vi "Defaults.vi"(8 "error in (no error)":errorcluster, 11 "MB Slave in":refnum<class "iC7-AFE.lvclass">) -> (0 "error out":errorcluster, 3 "MB Slave out":refnum<class "iC7-AFE.lvclass">)   [LabVIEW 2021, in "iC7-AFE.lvclass"]
uses:
  iC7-AFE.lvclass
  C:/Program Files (x86)/National Instruments/LabVIEW 2021/user.lib/S2 Labs/Module Framework/Modules/Base/Module.lvclass
  C:/Program Files (x86)/National Instruments/LabVIEW 2021/user.lib/S2 Labs/Module Framework/Modules/Modbus/Modbus Slave Base/Modbus Slave Base.lvclass
  <userlib>/S2 Labs/Module Framework/Modules/Base/Module.lvclass/Module.ctl
  <userlib>/S2 Labs/Modbus Toolkit/TypeDefs/MB Element.ctl
  <userlib>/S2 Labs/Modbus Toolkit/TypeDefs/Endianness Type.ctl
  <userlib>/S2 Labs/Modbus Toolkit/TypeDefs/Access Type.ctl
  <userlib>/S2 Labs/Module Framework/Modules/Modbus/Modbus Slave Base/Modbus Slave Base.lvclass/Modbus Slave Base.ctl
  <userlib>/S2 Labs/Module Framework/Modules/Base/Read Name.vi
  <userlib>/S2 Labs/Module Framework/Modules/Modbus/Modbus Slave Base/Write MB Map.vi
  MB Slave Simulator Base/MB Slave Simulator Base.lvclass
  <userlib>/S2 Labs/Modbus Toolkit/S2L Modbus API.lvclass
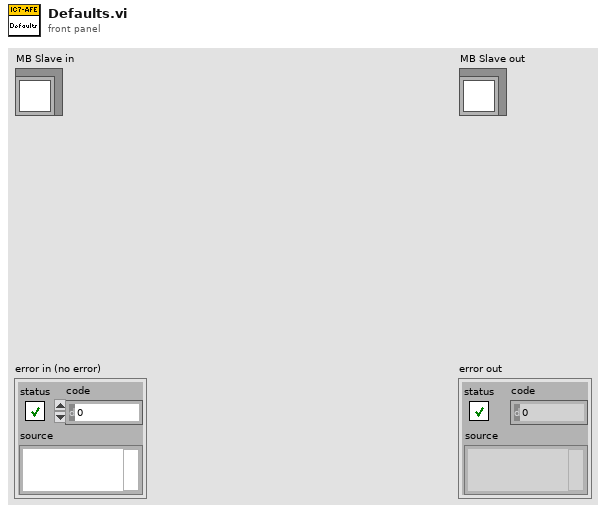
[diagram p1: front panel]
types:
  T1 = typedef "S2L Modbus API.lvclass/MB Element.ctl" = cluster{"Label":string, "Prefix":u8, "Address":u16, "Datatype":string, "Register Count":u8, "Multiplier":dbl, "Offset":dbl, "Unit":string, "Endianness":T2, "Access":T3, "LUT":string[], "Poll Rate(ms)":u16, "Mapping":cluster{"Module":string, "Channel":string}}
  T2 = typedef "Endianness Type.ctl" = enum16{"Big-Endian", "Little-Endian", "Big-Endian Byte Swap", "Little-Endian Byte Swap"}
  T3 = typedef "S2L Modbus API.lvclass/Access Type.ctl" = enum16{"R/W", "R", "W"}
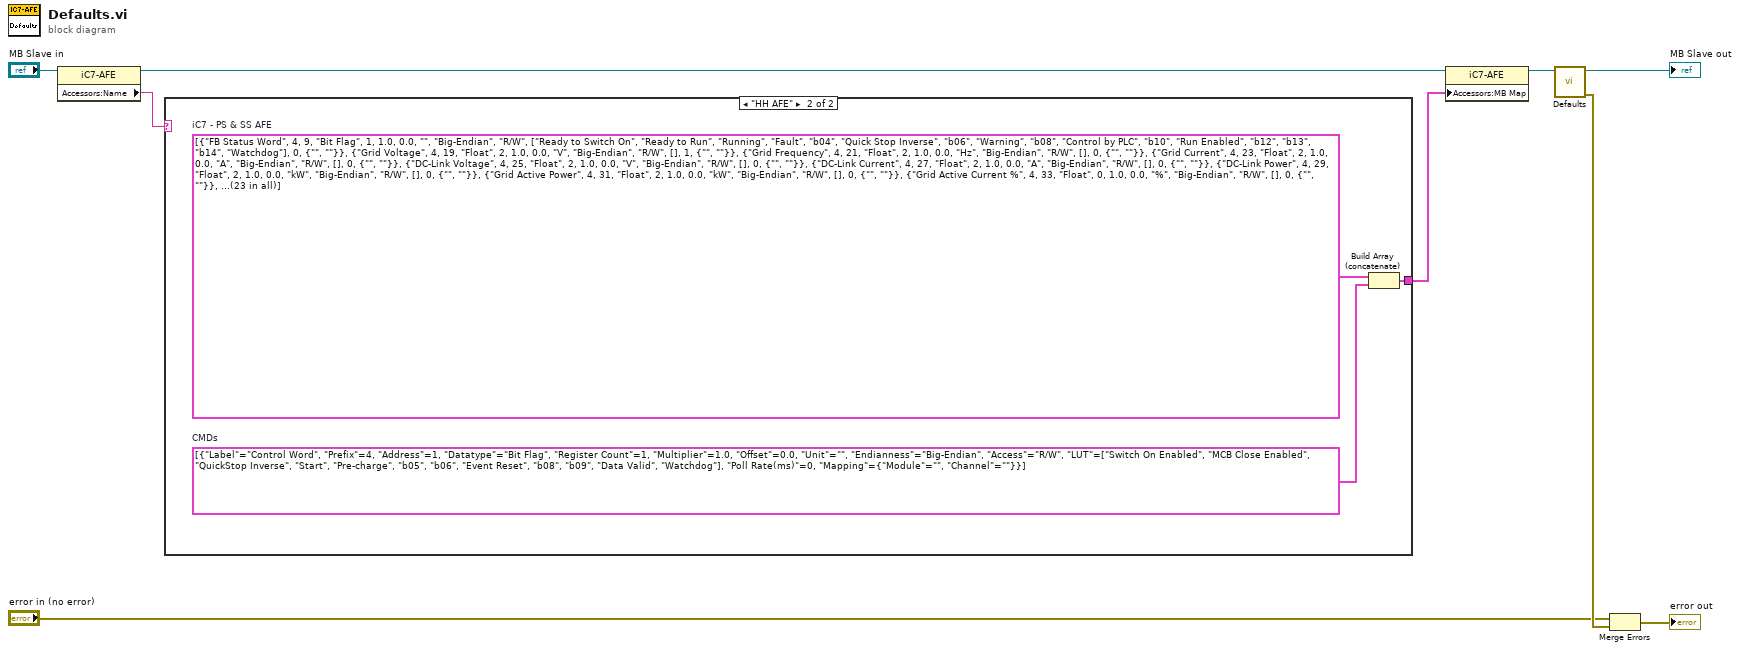
[diagram p0: block diagram]
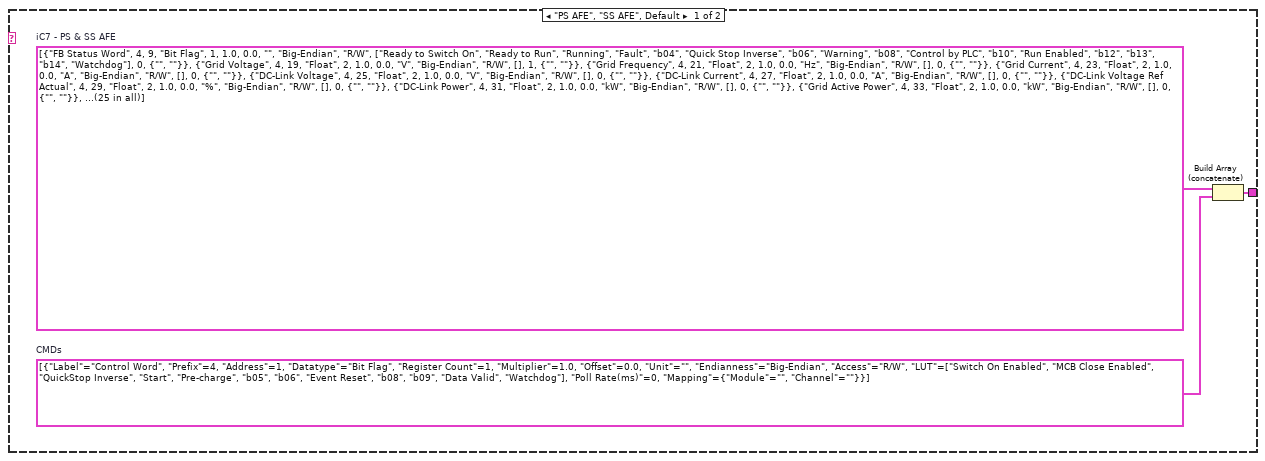
[diagram p2: hidden frame]
diagram:
  n1 = property class="iC7-AFE"(reference="MB Slave in") -> (reference out=w6:refnum<class "iC7-AFE.lvclass">, "Accessors:Name"=w1:string)  [unwired: 1 in, 1 out]
  n2 = case shown="\"HH AFE\"" w1 {
    tunnel: [w11 w14] -> w2
    frame "PS AFE", "SS AFE", Default {
      w10 = T1[] [{"Label"="Control Word", "Prefix"=4, "Address"=1, "Datatype"="Bit Flag", "Register Count"=1, "Multiplier"=1.0, "Offset"=0.0, "Unit"="", "Endianness"=enum."Big-Endian", "Access"=enum."R/W", "LUT"=["Switch On Enabled", "MCB Close Enabled", "QuickStop Inverse", "Start", "Pre-charge", "b05", "b06", "Event Reset", "b08", "b09", "Data Valid", "Watchdog"], "Poll Rate(ms)"=0, "Mapping"={"Module"="", "Channel"=""}}]  # CMDs
      w12 = T1[] [{"Label"="FB Status Word", "Prefix"=4, "Address"=9, "Datatype"="Bit Flag", "Register Count"=1, "Multiplier"=1.0, "Offset"=0.0, "Unit"="", "Endianness"=enum."Big-Endian", "Access"=enum."R/W", "LUT"=["Ready to Switch On", "Ready to Run", "Running", "Fault", "b04", "Quick Stop Inverse", "b06", "Warning", "b08", "Control by PLC", "b10", "Run Enabled", "b12", "b13", "b14", "Watchdog"], "Poll Rate(ms)"=0, "Mapping"={"Module"="", "Channel"=""}}, {"Label"="Grid Voltage", "Prefix"=4, "Address"=19, "Datatype"="Float", "Register Count"=2, "Multiplier"=1.0, "Offset"=0.0, "Unit"="V", "Endianness"=enum."Big-Endian", "Access"=enum."R/W", "LUT"=[], "Poll Rate(ms)"=1, "Mapping"={"Module"="", "Channel"=""}}, {"Label"="Grid Frequency", "Prefix"=4, "Address"=21, "Datatype"="Float", "Register Count"=2, "Multiplier"=1.0, "Offset"=0.0, "Unit"="Hz", "Endianness"=enum."Big-Endian", "Access"=enum."R/W", "LUT"=[], "Poll Rate(ms)"=0, "Mapping"={"Module"="", "Channel"=""}}, {"Label"="Grid Current", "Prefix"=4, "Address"=23, "Datatype"="Float", "Register Count"=2, "Multiplier"=1.0, "Offset"=0.0, "Unit"="A", "Endianness"=enum."Big-Endian", "Access"=enum."R/W", "LUT"=[], "Poll Rate(ms)"=0, "Mapping"={"Module"="", "Channel"=""}}, {"Label"="DC-Link Voltage", "Prefix"=4, "Address"=25, "Datatype"="Float", "Register Count"=2, "Multiplier"=1.0, "Offset"=0.0, "Unit"="V", "Endianness"=enum."Big-Endian", "Access"=enum."R/W", "LUT"=[], "Poll Rate(ms)"=0, "Mapping"={"Module"="", "Channel"=""}}, {"Label"="DC-Link Current", "Prefix"=4, "Address"=27, "Datatype"="Float", "Register Count"=2, "Multiplier"=1.0, "Offset"=0.0, "Unit"="A", "Endianness"=enum."Big-Endian", "Access"=enum."R/W", "LUT"=[], "Poll Rate(ms)"=0, "Mapping"={"Module"="", "Channel"=""}}, {"Label"="DC-Link Voltage Ref Actual", "Prefix"=4, "Address"=29, "Datatype"="Float", "Register Count"=2, "Multiplier"=1.0, "Offset"=0.0, "Unit"="%", "Endianness"=enum."Big-Endian", "Access"=enum."R/W", "LUT"=[], "Poll Rate(ms)"=0, "Mapping"={"Module"="", "Channel"=""}}, {"Label"="DC-Link Power", "Prefix"=4, "Address"=31, "Datatype"="Float", "Register Count"=2, "Multiplier"=1.0, "Offset"=0.0, "Unit"="kW", "Endianness"=enum."Big-Endian", "Access"=enum."R/W", "LUT"=[], "Poll Rate(ms)"=0, "Mapping"={"Module"="", "Channel"=""}}, {"Label"="Grid Active Power", "Prefix"=4, "Address"=33, "Datatype"="Float", "Register Count"=2, "Multiplier"=1.0, "Offset"=0.0, "Unit"="kW", "Endianness"=enum."Big-Endian", "Access"=enum."R/W", "LUT"=[], "Poll Rate(ms)"=0, "Mapping"={"Module"="", "Channel"=""}}, {"Label"="Grid Active Current %", "Prefix"=4, "Address"=35, "Datatype"="Float", "Register Count"=2, "Multiplier"=1.0, "Offset"=0.0, "Unit"="%", "Endianness"=enum."Big-Endian", "Access"=enum."R/W", "LUT"=[], "Poll Rate(ms)"=0, "Mapping"={"Module"="", "Channel"=""}}, {"Label"="Grid Reactive Current %", "Prefix"=4, "Address"=37, "Datatype"="Float", "Register Count"=2, "Multiplier"=1.0, "Offset"=0.0, "Unit"="%", "Endianness"=enum."Big-Endian", "Access"=enum."R/W", "LUT"=[], "Poll Rate(ms)"=0, "Mapping"={"Module"="", "Channel"=""}}, {"Label"="Grid Power Factor", "Prefix"=4, "Address"=39, "Datatype"="Float", "Register Count"=2, "Multiplier"=1.0, "Offset"=0.0, "Unit"="", "Endianness"=enum."Big-Endian", "Access"=enum."R/W", "LUT"=[], "Poll Rate(ms)"=0, "Mapping"={"Module"="", "Channel"=""}}, {"Label"="Fault Status Word 1", "Prefix"=4, "Address"=41, "Datatype"="Bit Flag", "Register Count"=1, "Multiplier"=1.0, "Offset"=0.0, "Unit"="", "Endianness"=enum."Big-Endian", "Access"=enum."R/W", "LUT"=["Over current", "DC-Link Over voltage", "DC-Link Under voltage", "b03-Reserved", "Unit under temperature", "b05-Reserved", "b06-Reserved", "b07-Reserved", "Earth Fault", "b09-Reserved", "Fieldbus issue", "HMI control lost", "b12-Reserved", "Thermistor Fault", "Auxiliary device", "External temperature measurement"], "Poll Rate(ms)"=0, "Mapping"={"Module"="", "Channel"=""}}, {"Label"="Fault Status Word 2", "Prefix"=4, "Address"=42, "Datatype"="Bit Flag", "Register Count"=1, "Multiplier"=1.0, "Offset"=0.0, "Unit"="", "Endianness"=enum."Big-Endian", "Access"=enum."R/W", "LUT"=["Analog Input Live Zero", "Pre charge Failed", "MCB Feedback Fault", "Quick Stop Active", "Thermistor Over Temperature", "MCB Trip", "External Fault", "Cooling Supervision Fault", "Fieldbus Watchdog", "Line Synchronization Fault", "Short Term Current Injection"], "Poll Rate(ms)"=0, "Mapping"={"Module"="", "Channel"=""}}, {"Label"="Warning Status Word 1", "Prefix"=4, "Address"=43, "Datatype"="Bit Flag", "Register Count"=1, "Multiplier"=1.0, "Offset"=0.0, "Unit"="", "Endianness"=enum."Big-Endian", "Access"=enum."R/W", "LUT"=["Over current", "DC-Link Over voltage", "DC-Link Under voltage", "b03-Reserved", "Unit under temperature ", "b05-Reserved", "b06-Reserved", "b07-Reserved", "Earth Warning", "b09-Reserved", "Fieldbus issue", "HMI control lost", "b12-Reserved", "Thermistor Warning", "Auxiliary device", "External temperature measurement"], "Poll Rate(ms)"=0, "Mapping"={"Module"="", "Channel"=""}}, {"Label"="Warning Status Word 2", "Prefix"=4, "Address"=44, "Datatype"="Bit Flag", "Register Count"=1, "Multiplier"=1.0, "Offset"=0.0, "Unit"="", "Endianness"=enum."Big-Endian", "Access"=enum."R/W", "LUT"=["Analog Input Live Zero", "b01-Reserved", "b02-Reserved", "Quick Stop Active", "Thermistor Over Temperature", "b05-Reserved", "External Warning", "Cooling Supervision Warning", "Fieldbus Watchdog", "b09-Reserved", "Short Term Current Injection"], "Poll Rate(ms)"=0, "Mapping"={"Module"="", "Channel"=""}}, {"Label"="DI Bit Word", "Prefix"=4, "Address"=45, "Datatype"="Bit Flag", "Register Count"=1, "Multiplier"=1.0, "Offset"=0.0, "Unit"="", "Endianness"=enum."Big-Endian", "Access"=enum."R/W", "LUT"=["b00", "b01", "b02", "Breaker Charged", "b04", "b05", "b06", "b07", "b08", "b09", "b10", "b11", "b12", "b13", "b14", "b15"], "Poll Rate(ms)"=0, "Mapping"={"Module"="", "Channel"=""}}, {"Label"="DO Bit Word", "Prefix"=4, "Address"=46, "Datatype"="Bit Flag", "Register Count"=1, "Multiplier"=1.0, "Offset"=0.0, "Unit"="", "Endianness"=enum."Big-Endian", "Access"=enum."R/W", "LUT"=["b00", "b01", "b02", "b03", "b04", "b05", "b06", "b07", "b08", "b09", "b10", "b11", "b12", "b13", "b14", "b15"], "Poll Rate(ms)"=0, "Mapping"={"Module"="", "Channel"=""}}, {"Label"="PreCharge Active", "Prefix"=4, "Address"=47, "Datatype"="U16", "Register Count"=1, "Multiplier"=1.0, "Offset"=0.0, "Unit"="", "Endianness"=enum."Big-Endian", "Access"=enum."R/W", "LUT"=[], "Poll Rate(ms)"=0, "Mapping"={"Module"="", "Channel"=""}}, {"Label"="MCB Feedback", "Prefix"=4, "Address"=48, "Datatype"="U16", "Register Count"=1, "Multiplier"=1.0, "Offset"=0.0, "Unit"="", "Endianness"=enum."Big-Endian", "Access"=enum."R/W", "LUT"=[], "Poll Rate(ms)"=0, "Mapping"={"Module"="", "Channel"=""}}, {"Label"="Heatsink Unit Temp", "Prefix"=4, "Address"=49, "Datatype"="Float", "Register Count"=2, "Multiplier"=1.0, "Offset"=0.0, "Unit"="C", "Endianness"=enum."Big-Endian", "Access"=enum."R/W", "LUT"=[], "Poll Rate(ms)"=0, "Mapping"={"Module"="", "Channel"=""}}, {"Label"="Grid Nominal Power", "Prefix"=4, "Address"=51, "Datatype"="Float", "Register Count"=2, "Multiplier"=1.0, "Offset"=0.0, "Unit"="kVA", "Endianness"=enum."Big-Endian", "Access"=enum."R/W", "LUT"=[], "Poll Rate(ms)"=0, "Mapping"={"Module"="", "Channel"=""}}, {"Label"="DC-Link Voltage Ref", "Prefix"=4, "Address"=53, "Datatype"="Float", "Register Count"=2, "Multiplier"=1.0, "Offset"=0.0, "Unit"="V", "Endianness"=enum."Big-Endian", "Access"=enum."R/W", "LUT"=[], "Poll Rate(ms)"=0, "Mapping"={"Module"="", "Channel"=""}}, {"Label"="DC-Link Voltage Ramp Rate", "Prefix"=4, "Address"=55, "Datatype"="Float", "Register Count"=2, "Multiplier"=1.0, "Offset"=0.0, "Unit"="percent/sec", "Endianness"=enum."Big-Endian", "Access"=enum."R/W", "LUT"=[], "Poll Rate(ms)"=0, "Mapping"={"Module"="", "Channel"=""}}, {"Label"="FB Active Power Ref", "Prefix"=4, "Address"=57, "Datatype"="Float", "Register Count"=2, "Multiplier"=1.0, "Offset"=0.0, "Unit"="kW", "Endianness"=enum."Big-Endian", "Access"=enum."R/W", "LUT"=[], "Poll Rate(ms)"=0, "Mapping"={"Module"="", "Channel"=""}}]  # iC7 - PS & SS AFE
      n3 = Build Array (concatenate)(w12, w10) -> (w11:T1[])
    }
    frame "HH AFE" {
      w13 = T1[] [{"Label"="Control Word", "Prefix"=4, "Address"=1, "Datatype"="Bit Flag", "Register Count"=1, "Multiplier"=1.0, "Offset"=0.0, "Unit"="", "Endianness"=enum."Big-Endian", "Access"=enum."R/W", "LUT"=["Switch On Enabled", "MCB Close Enabled", "QuickStop Inverse", "Start", "Pre-charge", "b05", "b06", "Event Reset", "b08", "b09", "Data Valid", "Watchdog"], "Poll Rate(ms)"=0, "Mapping"={"Module"="", "Channel"=""}}]  # CMDs
      w15 = T1[] [{"Label"="FB Status Word", "Prefix"=4, "Address"=9, "Datatype"="Bit Flag", "Register Count"=1, "Multiplier"=1.0, "Offset"=0.0, "Unit"="", "Endianness"=enum."Big-Endian", "Access"=enum."R/W", "LUT"=["Ready to Switch On", "Ready to Run", "Running", "Fault", "b04", "Quick Stop Inverse", "b06", "Warning", "b08", "Control by PLC", "b10", "Run Enabled", "b12", "b13", "b14", "Watchdog"], "Poll Rate(ms)"=0, "Mapping"={"Module"="", "Channel"=""}}, {"Label"="Grid Voltage", "Prefix"=4, "Address"=19, "Datatype"="Float", "Register Count"=2, "Multiplier"=1.0, "Offset"=0.0, "Unit"="V", "Endianness"=enum."Big-Endian", "Access"=enum."R/W", "LUT"=[], "Poll Rate(ms)"=1, "Mapping"={"Module"="", "Channel"=""}}, {"Label"="Grid Frequency", "Prefix"=4, "Address"=21, "Datatype"="Float", "Register Count"=2, "Multiplier"=1.0, "Offset"=0.0, "Unit"="Hz", "Endianness"=enum."Big-Endian", "Access"=enum."R/W", "LUT"=[], "Poll Rate(ms)"=0, "Mapping"={"Module"="", "Channel"=""}}, {"Label"="Grid Current", "Prefix"=4, "Address"=23, "Datatype"="Float", "Register Count"=2, "Multiplier"=1.0, "Offset"=0.0, "Unit"="A", "Endianness"=enum."Big-Endian", "Access"=enum."R/W", "LUT"=[], "Poll Rate(ms)"=0, "Mapping"={"Module"="", "Channel"=""}}, {"Label"="DC-Link Voltage", "Prefix"=4, "Address"=25, "Datatype"="Float", "Register Count"=2, "Multiplier"=1.0, "Offset"=0.0, "Unit"="V", "Endianness"=enum."Big-Endian", "Access"=enum."R/W", "LUT"=[], "Poll Rate(ms)"=0, "Mapping"={"Module"="", "Channel"=""}}, {"Label"="DC-Link Current", "Prefix"=4, "Address"=27, "Datatype"="Float", "Register Count"=2, "Multiplier"=1.0, "Offset"=0.0, "Unit"="A", "Endianness"=enum."Big-Endian", "Access"=enum."R/W", "LUT"=[], "Poll Rate(ms)"=0, "Mapping"={"Module"="", "Channel"=""}}, {"Label"="DC-Link Power", "Prefix"=4, "Address"=29, "Datatype"="Float", "Register Count"=2, "Multiplier"=1.0, "Offset"=0.0, "Unit"="kW", "Endianness"=enum."Big-Endian", "Access"=enum."R/W", "LUT"=[], "Poll Rate(ms)"=0, "Mapping"={"Module"="", "Channel"=""}}, {"Label"="Grid Active Power", "Prefix"=4, "Address"=31, "Datatype"="Float", "Register Count"=2, "Multiplier"=1.0, "Offset"=0.0, "Unit"="kW", "Endianness"=enum."Big-Endian", "Access"=enum."R/W", "LUT"=[], "Poll Rate(ms)"=0, "Mapping"={"Module"="", "Channel"=""}}, {"Label"="Grid Active Current %", "Prefix"=4, "Address"=33, "Datatype"="Float", "Register Count"=0, "Multiplier"=1.0, "Offset"=0.0, "Unit"="%", "Endianness"=enum."Big-Endian", "Access"=enum."R/W", "LUT"=[], "Poll Rate(ms)"=0, "Mapping"={"Module"="", "Channel"=""}}, {"Label"="Grid Reactive Current %", "Prefix"=4, "Address"=35, "Datatype"="Float", "Register Count"=0, "Multiplier"=1.0, "Offset"=0.0, "Unit"="%", "Endianness"=enum."Big-Endian", "Access"=enum."R/W", "LUT"=[], "Poll Rate(ms)"=0, "Mapping"={"Module"="", "Channel"=""}}, {"Label"="Grid Power Factor", "Prefix"=4, "Address"=37, "Datatype"="Float", "Register Count"=0, "Multiplier"=1.0, "Offset"=0.0, "Unit"="", "Endianness"=enum."Big-Endian", "Access"=enum."R/W", "LUT"=[], "Poll Rate(ms)"=0, "Mapping"={"Module"="", "Channel"=""}}, {"Label"="Fault Status Word 1", "Prefix"=4, "Address"=39, "Datatype"="Bit Flag", "Register Count"=0, "Multiplier"=1.0, "Offset"=0.0, "Unit"="", "Endianness"=enum."Big-Endian", "Access"=enum."R/W", "LUT"=["Over current", "DC-Link Over voltage", "DC-Link Under voltage", "b03-Reserved", "Unit under temperature", "b05-Reserved", "b06-Reserved", "b07-Reserved", "Earth Fault", "b09-Reserved", "Fieldbus issue", "HMI control lost", "b12-Reserved", "Thermistor Fault", "Auxiliary device", "External temperature measurement"], "Poll Rate(ms)"=0, "Mapping"={"Module"="", "Channel"=""}}, {"Label"="Fault Status Word 2", "Prefix"=4, "Address"=40, "Datatype"="Bit Flag", "Register Count"=0, "Multiplier"=1.0, "Offset"=0.0, "Unit"="", "Endianness"=enum."Big-Endian", "Access"=enum."R/W", "LUT"=["Analog Input Live Zero", "Pre charge Failed", "MCB Feedback Fault", "Quick Stop Active", "Thermistor Over Temperature", "MCB Trip", "External Fault", "Cooling Supervision Fault", "Fieldbus Watchdog", "Line Synchronization Fault", "Short Term Current Injection"], "Poll Rate(ms)"=0, "Mapping"={"Module"="", "Channel"=""}}, {"Label"="Warning Status Word 1", "Prefix"=4, "Address"=41, "Datatype"="Bit Flag", "Register Count"=0, "Multiplier"=1.0, "Offset"=0.0, "Unit"="", "Endianness"=enum."Big-Endian", "Access"=enum."R/W", "LUT"=["Over current", "DC-Link Over voltage", "DC-Link Under voltage", "b03-Reserved", "Unit under temperature ", "b05-Reserved", "b06-Reserved", "b07-Reserved", "Earth Warning", "b09-Reserved", "Fieldbus issue", "HMI control lost", "b12-Reserved", "Thermistor Warning", "Auxiliary device", "External temperature measurement"], "Poll Rate(ms)"=0, "Mapping"={"Module"="", "Channel"=""}}, {"Label"="Warning Status Word 2", "Prefix"=4, "Address"=42, "Datatype"="Bit Flag", "Register Count"=0, "Multiplier"=1.0, "Offset"=0.0, "Unit"="", "Endianness"=enum."Big-Endian", "Access"=enum."R/W", "LUT"=["Analog Input Live Zero", "b01-Reserved", "b02-Reserved", "Quick Stop Active", "Thermistor Over Temperature", "b05-Reserved", "External Warning", "Cooling Supervision Warning", "Fieldbus Watchdog", "b09-Reserved", "Short Term Current Injection"], "Poll Rate(ms)"=0, "Mapping"={"Module"="", "Channel"=""}}, {"Label"="DI Bit Word", "Prefix"=4, "Address"=43, "Datatype"="Bit Flag", "Register Count"=0, "Multiplier"=1.0, "Offset"=0.0, "Unit"="", "Endianness"=enum."Big-Endian", "Access"=enum."R/W", "LUT"=["b00", "b01", "b02", "b03", "b04", "b05", "b06", "b07", "b08", "b09", "b10", "b11", "b12", "b13", "b14", "b15"], "Poll Rate(ms)"=0, "Mapping"={"Module"="", "Channel"=""}}, {"Label"="DO Bit Word", "Prefix"=4, "Address"=44, "Datatype"="Bit Flag", "Register Count"=0, "Multiplier"=1.0, "Offset"=0.0, "Unit"="", "Endianness"=enum."Big-Endian", "Access"=enum."R/W", "LUT"=["b00", "b01", "b02", "b03", "b04", "b05", "b06", "b07", "b08", "b09", "b10", "b11", "b12", "b13", "b14", "b15"], "Poll Rate(ms)"=0, "Mapping"={"Module"="", "Channel"=""}}, {"Label"="PreCharge Active", "Prefix"=4, "Address"=45, "Datatype"="U16", "Register Count"=0, "Multiplier"=1.0, "Offset"=0.0, "Unit"="", "Endianness"=enum."Big-Endian", "Access"=enum."R/W", "LUT"=[], "Poll Rate(ms)"=0, "Mapping"={"Module"="", "Channel"=""}}, {"Label"="MCB Feedback", "Prefix"=4, "Address"=46, "Datatype"="U16", "Register Count"=0, "Multiplier"=1.0, "Offset"=0.0, "Unit"="", "Endianness"=enum."Big-Endian", "Access"=enum."R/W", "LUT"=[], "Poll Rate(ms)"=0, "Mapping"={"Module"="", "Channel"=""}}, {"Label"="Heatsink Unit Temp", "Prefix"=4, "Address"=47, "Datatype"="Float", "Register Count"=0, "Multiplier"=1.0, "Offset"=0.0, "Unit"="C", "Endianness"=enum."Big-Endian", "Access"=enum."R/W", "LUT"=[], "Poll Rate(ms)"=0, "Mapping"={"Module"="", "Channel"=""}}, {"Label"="Grid Nominal Power", "Prefix"=4, "Address"=49, "Datatype"="Float", "Register Count"=0, "Multiplier"=1.0, "Offset"=0.0, "Unit"="kVA", "Endianness"=enum."Big-Endian", "Access"=enum."R/W", "LUT"=[], "Poll Rate(ms)"=0, "Mapping"={"Module"="", "Channel"=""}}, {"Label"="DC-Link Voltage Ref", "Prefix"=4, "Address"=51, "Datatype"="Float", "Register Count"=0, "Multiplier"=1.0, "Offset"=0.0, "Unit"="V", "Endianness"=enum."Big-Endian", "Access"=enum."R/W", "LUT"=[], "Poll Rate(ms)"=0, "Mapping"={"Module"="", "Channel"=""}}, {"Label"="FB Active Power Ref", "Prefix"=4, "Address"=53, "Datatype"="Float", "Register Count"=0, "Multiplier"=1.0, "Offset"=0.0, "Unit"="kW", "Endianness"=enum."Big-Endian", "Access"=enum."R/W", "LUT"=[], "Poll Rate(ms)"=0, "Mapping"={"Module"="", "Channel"=""}}]  # iC7 - PS & SS AFE
      n4 = Build Array (concatenate)(w15, w13) -> (w14:T1[])
    }
  }
  n5 = property class="iC7-AFE"(reference=w6, "Accessors:MB Map"=w2) -> (reference out=w5:refnum<class "iC7-AFE.lvclass">)  [unwired: 1 in, 1 out]
  n6 = call-parent "Defaults.vi"("MB Slave in"=w5) -> ("error out"=w9:errorcluster, "MB Slave out"=→"MB Slave out":refnum<class "iC7-AFE.lvclass">)  [unwired: 9 in]
  n7 = Merge Errors("error in (no error)", w9) -> (→"error out":errorcluster)
